vi "Prism_Checksum.vi"(10 "ID +DB+ Data":string) -> (1 "Full Cmd":string)   [LabVIEW 2020]
panel:
  out "ID +DB+ Data 2":string
  out "Chksum only":string
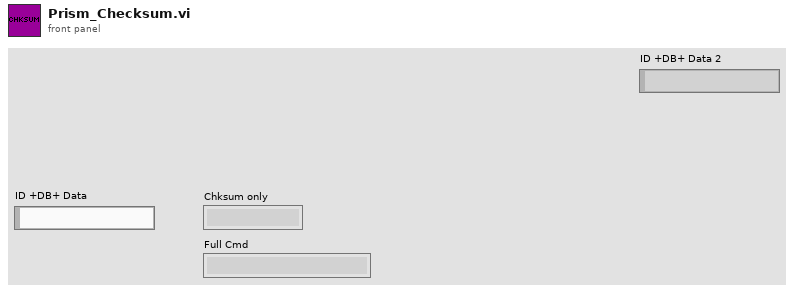
[diagram p1: front panel]
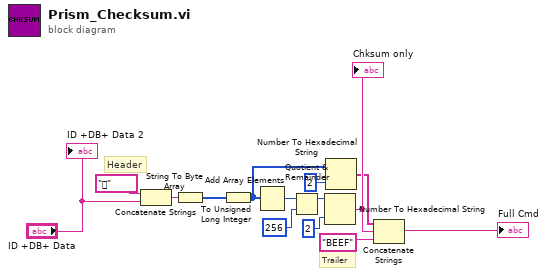
[diagram p0: block diagram]
diagram:
  # "Trailer"
  # "Header"
  n1 = Concatenate Strings("ޭ" ("string"), "ID +DB+ Data") -> (w8:string)
  n2 = String To Byte Array(string=w8) -> (unsigned byte array=w14:u8[])
  n3 = To Unsigned Long Integer(number=w14) -> (unsigned 32bit integer=w2:u32[])
  n4 = Add Array Elements(numeric array=w2) -> (sum=w6:u32)
  n5 = Quotient & Remainder(x=w6, y=u32 256) -> (x-y*floor(x/y)=w11:u32)  [unwired: 1 out]
  n6 = Number To Hexadecimal String(1:i16 2 ("width (-)"), 2:w11) -> (0:w10:string)
  "Chksum only" <- w10
  n7 = Number To Hexadecimal String(1:i16 2 ("width (-)"), 2:w2) -> (0:w4:string[])
  n8 = Concatenate Strings(w4, w10, "BEEF" ("string")) -> (→"Full Cmd":string)
  "ID +DB+ Data 2" <- "ID +DB+ Data"
